vi "lib Add Error Text.vi"(8 "error in (no error)":errorcluster, 11 "Append to source, if error":string) -> (0 "error out":errorcluster)   [LabVIEW 2024]
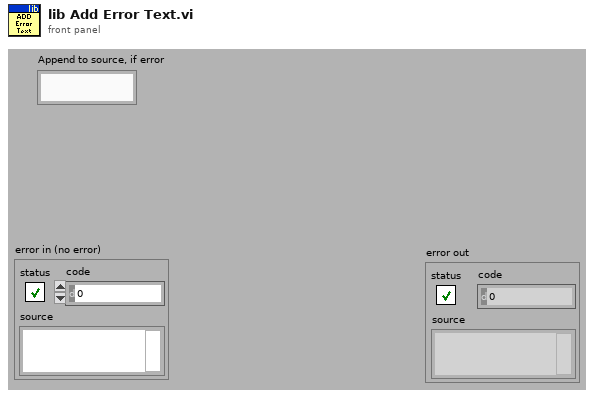
[diagram p1: front panel]
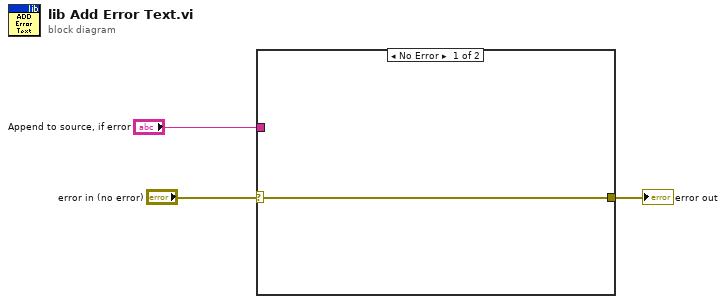
[diagram p0: block diagram]
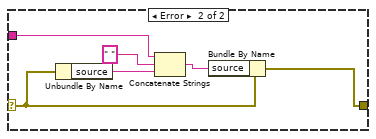
[diagram p2: hidden frame]
diagram:
  n1 = case shown="No Error" "error in (no error)" {
    selector: "error in (no error)" -> [w4 w7]
    tunnel: "Append to source, if error" -> [_ w9]
    tunnel: [w4 w5] -> w1
    frame No Error {
    }
    frame Error {
      n2 = Unbundle By Name(w7) -> ("source"=w10:string)
      n3 = Concatenate Strings(w9, " " ("string"), w10) -> (w6:string)
      n4 = Bundle By Name(cluster=w7, "source"=w6) -> (w5:errorcluster)
    }
  }
  "error out" <- w1
